vi "Install Software To Target if Not Installed.vi"(7 "Install (T)":bool=TRUE, 8 "error in (no error)":errorcluster, 11 "MAC Address":string) -> (0 "error out":errorcluster, 4 "Installed":bool)   [LabVIEW 2013]
uses:
  <vilib>/nisyscfg/Get Available Components.vi
  <vilib>/nisyscfg/Get Installed Components.vi
  <vilib>/nisyscfg/Close (System).vi
  <vilib>/nisyscfg/Install or Uninstall Components.vi
  <vilib>/nisyscfg/nisyscfg.lvlib
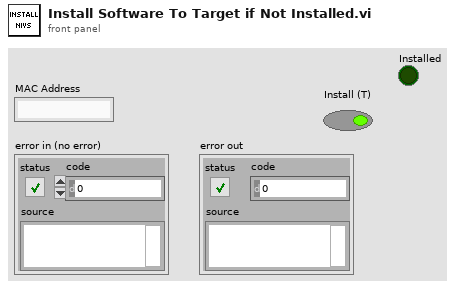
[diagram p1: front panel]
types:
  T1 = typedef "nisyscfg.lvlib/Software 1.2.ctl" = cluster{"title":string, "description":string, "ID":string, "version":string, "component type":T2}
  T2 = typedef "nisyscfg.lvlib/Component Type.ctl" = u32
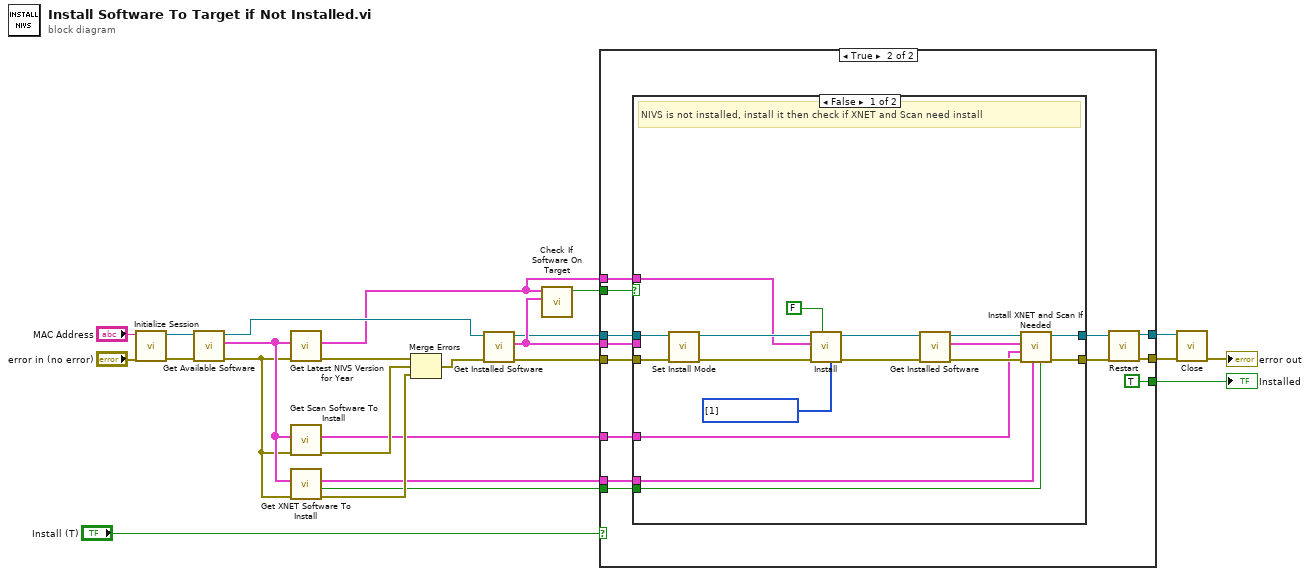
[diagram p0: block diagram]
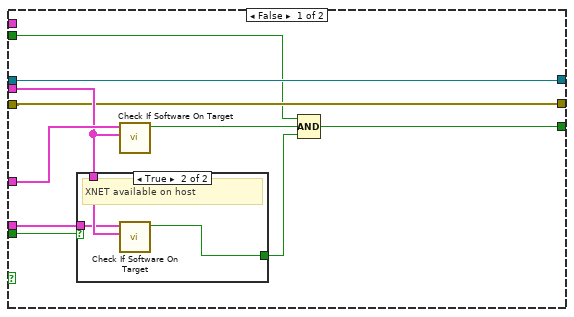
[diagram p2: hidden frame]
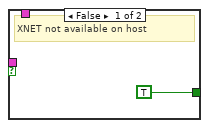
[diagram p3: hidden frame]
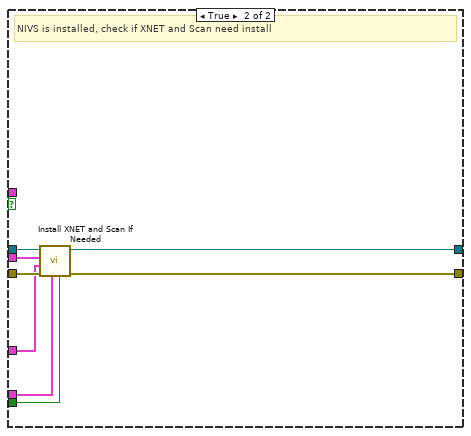
[diagram p4: hidden frame]
diagram:
  n1 = call <vilib>:"Initialize Session.vi"("error in (no error)"="error in (no error)", "target (localhost)"="MAC Address") -> ("error out"=w21:errorcluster, "session out"=w20:refnum<k21>)  [unwired: 8 in]
  n2 = call-poly <vilib>:"Get Available Software.vi"("error in (no error)"=w21, "session in"=w20) -> ("error out"=w18:errorcluster, "software components"=w19:T1[], "session out"=w8:refnum<k21>)  [unwired: 7 in]
  n3 = call "Get Latest NIVS Version for Year.vi"("error in (no error)"=w18, "software components"=w19) -> ("error out"=w17:errorcluster, "nivs software to install"=w3:T1[])  [unwired: 7 in, 1 out]
  n4 = call "Get Scan Software To Install.vi"("error in (no error)"=w18, "available software components"=w19) -> ("error out"=w16:errorcluster, "scan software to install"=w4:T1[])  [unwired: 7 in, 1 out]
  n5 = call "Get XNET Software To Install.vi"("error in (no error)"=w18, "available software components"=w19) -> ("error out"=w15:errorcluster, "found"=w11:bool, "xnet software to install"=w9:T1[])  [unwired: 7 in]
  n6 = Merge Errors(w17, w16, w15) -> (w14:errorcluster)
  n7 = call-poly <vilib>:"Get Installed Software.vi"("error in (no error)"=w14, "session in"=w8) -> ("error out"=w12:errorcluster, "software components"=w10:T1[], "session out"=w7:refnum<k21>)  [unwired: 7 in]
  n8 = call "Check If Software On Target.vi"("installed software"=w10, "software to check"=w3) -> ("software installed"=w13:bool)  [unwired: 8 in, 1 out]
  n9 = case shown="True" "Install (T)" {
    tunnel: w13 -> [w29 w51]
    tunnel: w12 -> [w30 w50]
    tunnel: w11 -> [w32 w49]
    tunnel: w10 -> [w33 w48]
    tunnel: w9 -> [w26 w47]
    tunnel: w7 -> [w31 w46]
    tunnel: [w30 w45] -> w6
    tunnel: [w31 w44] -> w5
    tunnel: w4 -> [w34 w41]
    tunnel: w3 -> [_ w40]
    tunnel: [w25 TRUE] -> w1
    frame False {
      n10 = case shown="True" w32 {
        tunnel: w33 -> [_ w38]
        tunnel: [TRUE w37] -> w27
        tunnel: w26 -> [_ w36]
        frame False {
          # "XNET not available on host"
        }
        frame True {
          # "XNET available on host"
          n11 = call "Check If Software On Target.vi"("installed software"=w38, "software to check"=w36) -> ("software installed"=w37:bool)  [unwired: 8 in, 1 out]
        }
      }
      n12 = call "Check If Software On Target.vi"("installed software"=w33, "software to check"=w34) -> ("software installed"=w28:bool)  [unwired: 8 in, 1 out]
      n13 = Compound Arithmetic op=AND(w29, w28, w27) -> (w25:bool)
    }
    frame True {
      n14 = case shown="False" w51 {
        tunnel: w50 -> [w68 w76]
        tunnel: w49 -> [w56 w70]
        tunnel: w48 -> [_ w72]
        tunnel: w47 -> [w55 w71]
        tunnel: w46 -> [w67 w75]
        tunnel: [w53 w74] -> w43
        tunnel: [w52 w73] -> w42
        tunnel: w41 -> [w54 w69]
        tunnel: w40 -> [w62 _]
        frame False {
          w66 = u32[] [1] items=["Highest", "Exactly"] ("version selection (highest)")
          # "NIVS is not installed, install it then check if XNET and Scan need install"
          n15 = call "Set Install Mode.vi"("error in"=w68, "session in"=w67) -> ("error out"=w64:errorcluster, "session out"=w63:refnum<k21>)  [unwired: 8 in]
          n16 = call-poly <vilib>:"Install.vi"("version selection (highest)"=w66, "restart automatically (T)"=FALSE, "error in (no error)"=w64, "software components to install"=w62, "session in"=w63) -> ("error out"=w61:errorcluster, "session out"=w60:refnum<k21>)  [unwired: 4 in, 1 out]
          n17 = call-poly <vilib>:"Get Installed Software.vi"("error in (no error)"=w61, "session in"=w60) -> ("error out"=w59:errorcluster, "software components"=w57:T1[], "session out"=w58:refnum<k21>)  [unwired: 7 in]
          n18 = call "Install XNET and Scan If Needed.vi"("XNET available"=w56, "xnet software to install"=w55, "error in (no error)"=w59, "scan software to install"=w54, "software components on target"=w57, "Refnum in"=w58) -> ("error out"=w53:errorcluster, "Refnum out"=w52:refnum<k21>)  [unwired: 4 in]
        }
        frame True {
          # "NIVS is installed, check if XNET and Scan need install"
          n19 = call "Install XNET and Scan If Needed.vi"("XNET available"=w70, "xnet software to install"=w71, "error in (no error)"=w76, "scan software to install"=w69, "software components on target"=w72, "Refnum in"=w75) -> ("error out"=w74:errorcluster, "Refnum out"=w73:refnum<k21>)  [unwired: 4 in]
        }
      }
      n20 = call <vilib>:"Restart.vi"("error in (no error)"=w43, "session in"=w42) -> ("error out"=w45:errorcluster, "session out"=w44:refnum<k21>)  [unwired: 7 in, 1 out]
    }
  }
  "Installed" <- w1
  n21 = call-poly <vilib>:"Close.vi"("error in (no error)"=w6, "session in"=w5) -> ("error out"=→"error out":errorcluster)  [unwired: 9 in]
